vi "Komunikat.vi"(1 "String 2":string) -> (0 "OUT":bool)   [LabVIEW 2019]
panel:
  in  "CANCEL":bool
  in  "OK":bool
  out "String":string
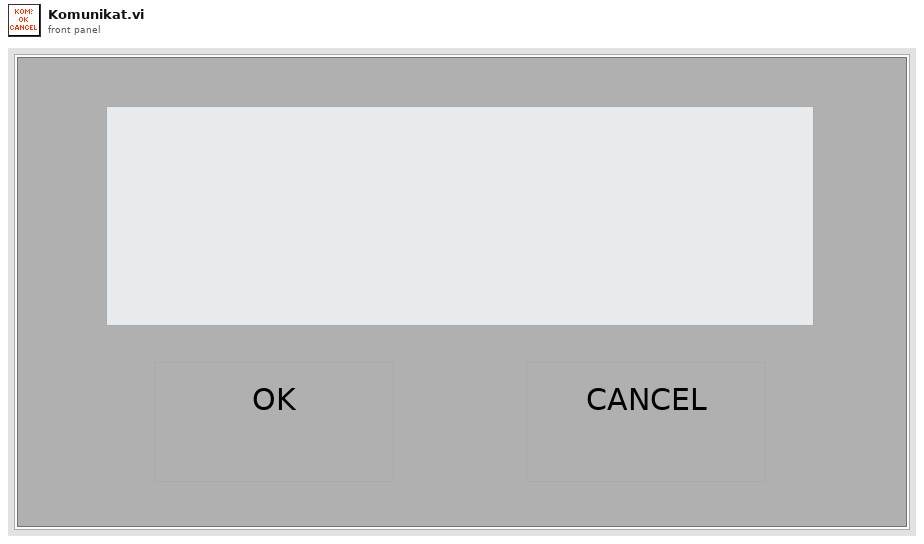
[diagram p1: front panel]
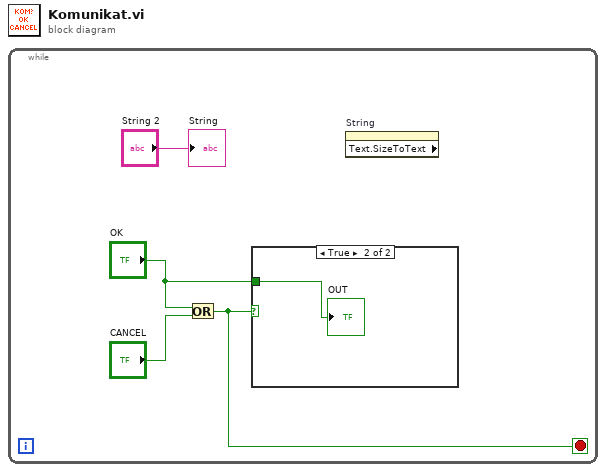
[diagram p0: block diagram]
diagram:
  n1 = while {
    stop <- w2 stop-if-true
    n2 = Or(x="OK", y="CANCEL") -> (x .or. y?=w2:bool)
    n3 = case shown="True" w2 {
      tunnel: "OK" -> [_ w5]
      frame False {
      }
      frame True {
        "OUT" <- w5
      }
    }
    n4 = property on="String" class="Str" props=["Text", "SizeToText"]() -> ()  [unwired: 2 in, 3 out]
    "String" <- "String 2"
  }
